vi "Get Pin Object.vi"   [LabVIEW 2021, in "DMM_Base.lvclass"]
doc: "This polymorphic VI gets the `session reservation` and either a single or an array of base class instrument objects from `pin or relay name(s)`."
uses:
  DMM_Base.lvclass
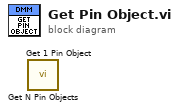
[diagram p0: block diagram]
diagram:
  n1 = call "Get N Pin Objects.vi"() -> ()  [unwired: 9 in, 3 out]
  n2 = call "Get 1 Pin Object.vi"() -> ()  [unwired: 9 in, 3 out]
